vi "Teleop.vi"(10 "Match Info":T2={"Autonomous Elapsed Seconds"=0.0, "TeleOp Elapsed Seconds"=0.0, "Disabled Elapsed Seconds"=0.0, "Visited Autonomous"=FALSE, "Visited TeleOp"=FALSE, "Visited Disabled"=FALSE, "Autonomous Settings"={"Autonomous Style"=enum."Independent", "VI Refnum"=refnum}}, 11 "Call Context":T3) -> ()   [LabVIEW 2014]
doc: "This VI is called for each TeleOp packet received from the DS where the robot is not disabled. It is often used to read from the joysticks and update I/O or to update setpoints for timed control loops. It should complete and return within 20 milliseconds or it may miss DS packets."
uses:
  <vilib>/Rock Robotics/WPI/DriverStation/WPI_DriverStationDerivedRobotMode.ctl
  <vilib>/Rock Robotics/WPI/DriverStation/WPI_DriverStationMatch Info.ctl
  <vilib>/Rock Robotics/WPI/Joystick/WPI_JoystickGetSetRefNum.vi
  <vilib>/Rock Robotics/Network Tables/SD Write Boolean.vi
  <vilib>/Rock Robotics/Network Tables/SD Write Numeric Array.vi
  <vilib>/Rock Robotics/Network Tables/SD Read Boolean.vi
  <vilib>/Rock Robotics/Network Tables/SD Read Number.vi
  <vilib>/Utility/file.llb/Write To Spreadsheet File (DBL).vi
  <vilib>/Rock Robotics/WPI/RobotDrive/WPI_RobotDriveGetSetRefNum.vi
  <vilib>/Rock Robotics/WPI/RobotDrive/WPI_RobotDriveArcadeDrive_Standard(NoSaturation).vi
panel:
  in  "Claw Opened Limit":bool
  in  "Claw Closed Limit":bool
  in  "Bottom Limit":bool
  in  "Top Limit":bool
  in  "Button b":bool
  in  "Button a":bool
  in  "point reached":bool
  out "Time For Manipulator":dbl
  in  "Button y":bool
  in  "Button x":bool
  in  "Manipulator State":T1(ring)
  out "error out 2":errorcluster
  out "current (A)":dbl
  out "all currents (A)":dbl[](array[numeric])
  out "Power (W)":dbl
  out "error out 5":errorcluster
  out "error out":errorcluster
  out "Motor Values":dbl[](array[numeric])
  out "Buttons":bool[](array[boolean])
  out "Sample Slider 0":dbl(slide) scale=0.0..5.0
  out "Sample Boolean 1":bool
  out "Sample Boolean 0":bool
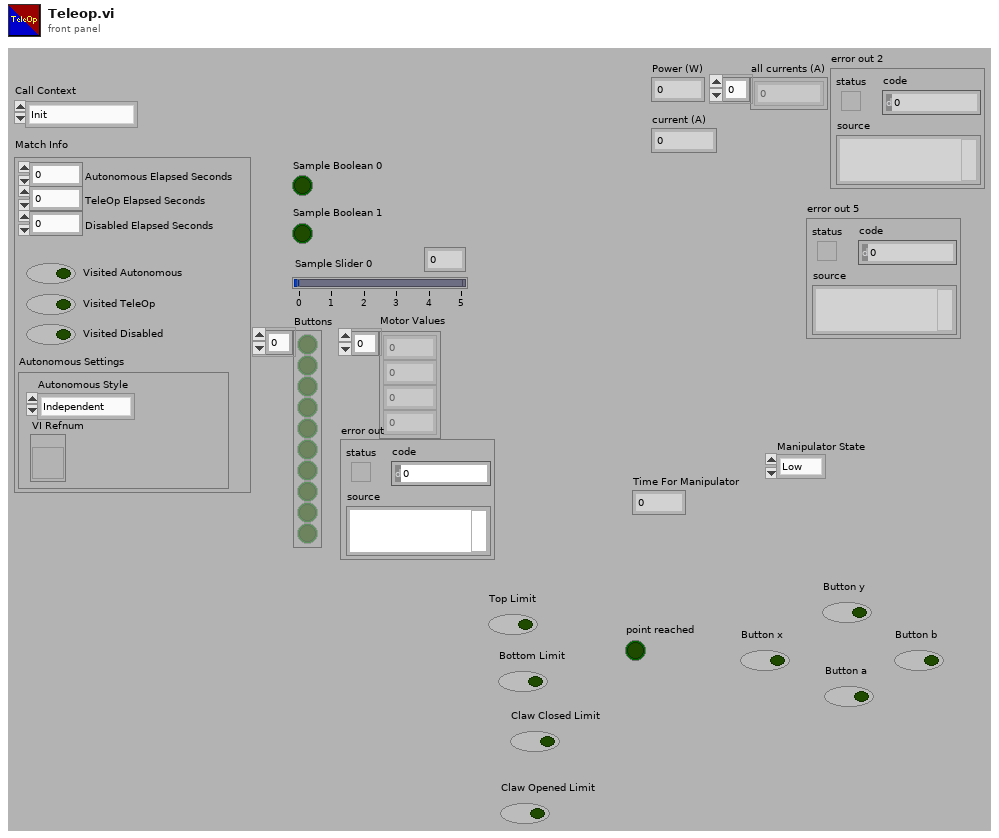
[diagram p1: front panel]
types:
  T1 = enum16{"Low", "RC Close", "Tote Close", "RC High", "Tote High", "Lowering", "Opening", "RC Top Stacker", "Bottom Stacking", "RC raising", "Tote Raising", "Limit High"}
  T2 = typedef "WPI_DriverStationMatch Info.ctl" = cluster{"Autonomous Elapsed Seconds":dbl, "TeleOp Elapsed Seconds":dbl, "Disabled Elapsed Seconds":dbl, "Visited Autonomous":bool, "Visited TeleOp":bool, "Visited Disabled":bool, "Autonomous Settings":cluster{"Autonomous Style":enum16{"Iterative", "Independent"}, "VI Refnum":refnum<vi>}}
  T3 = typedef "WPI_DriverStationDerivedRobotMode.ctl" = enum16{"Init", "Execute", "Stop"}
  T4 = typedef "WPI_RobotDriveDevRef.ctl" = cluster{"DevStatus":errorcluster, "Motors[]":T5[], "Square Inputs":bool, "Max Output":dbl}
  T5 = typedef "WPI_MotorControlDeviceRef.ctl" = cluster{"DeviceStatus":errorcluster, "Type":T6, "PWM":cluster{"Controller":T7, "PWM Channel":T8, "DeadBand":T9}, "CAN":cluster{"Device Number":u8, "Control Mode":T10, "Semaphore":T11, "Max Vout":dbl, "TalonSRX Control Mode":T12}, "Invert":bool, "TransformRef":T13, "InvTransformRef":T13}
  T6 = typedef "WPI_MotorControlType.ctl" = enum16{"PWM", "CAN", "CANTalonSRX"}
  T7 = typedef "FPGA_TypedefDigitalModule.ctl" = enum16{"Controller 1"}
  T8 = typedef "FPGA_DIOPWMChannel.ctl" = enum8{"PWM 0", "PWM 1", "PWM 2", "PWM 3", "PWM 4", "PWM 5", "PWM 6", "PWM 7", "PWM 8", "PWM 9", "PWM MXP 0", "PWM MXP 1", "PWM MXP 2", "PWM MXP 3", "PWM MXP 4", "PWM MXP 5", "PWM MXP 6", "PWM MXP 7", "PWM MXP 8", "PWM MXP 9", "Invalid"}
  T9 = typedef "WPI_PWMDeadband.ctl" = cluster{"Name":string, "maxPositivePwm":i32, "minPositivePwm":i32, "centerPwm":i32, "maxNegativePwm":i32, "minNegativePwm":i32, "angularRange":u16}
  T10 = typedef "WPI_CANJaguar_ControlMode.ctl" = enum8{"Percent VBus", "Current", "Speed", "Position", "Voltage"}
  T11 = typedef "Semaphore RefNum" = refnum<k1>
  T12 = typedef "WPI_CANTalonSRX_APIControlMode.ctl" = enum8{"Percent VBus", "Speed", "Position", "Slave", "Unchanged / Invalid"}
  T13 = typedef "WPI_PWMTransform_ConPane.ctl" = refnum<vi>
  T14 = typedef "WPI_JoystickDevRef.ctl" = cluster{"Device":T15}
  T15 = typedef "WPI_JoystickDeviceEnum.ctl" = enum16{"USB 0", "USB 1", "USB 2", "USB 3", "USB 4", "USB 5"}
  T16 = enum16{"Low", "RC Close", "Tote Close", "RC High", "Tote High", "Lowering", "Opening", "RC Top Stacker", "Bottom Stacking"}
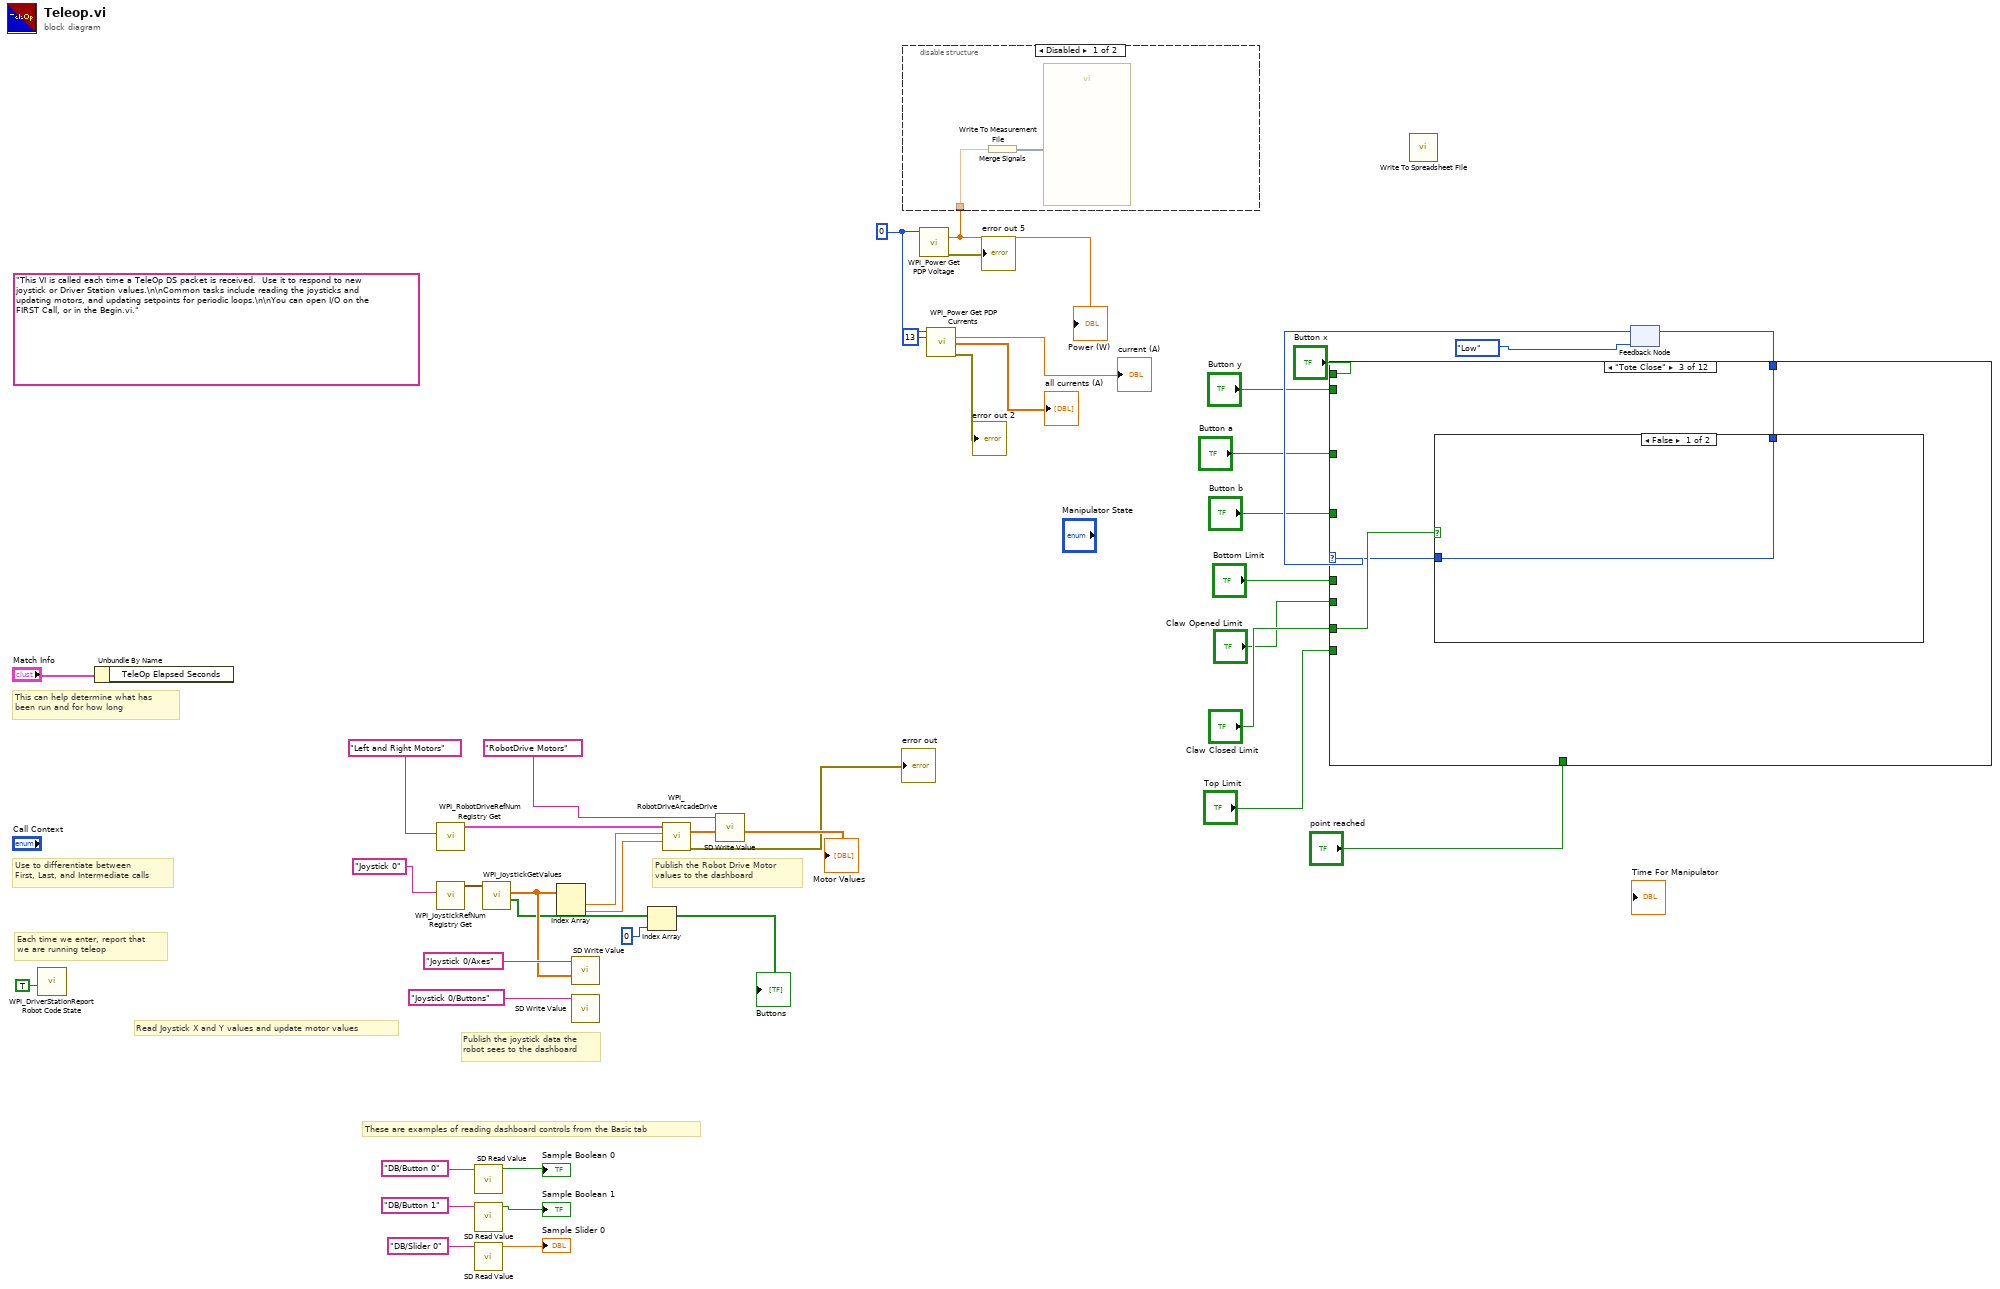
[diagram p0: block diagram]
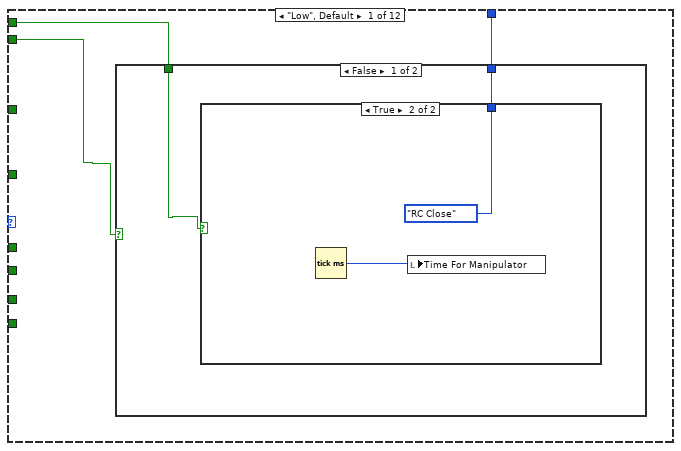
[diagram p2: hidden frame]
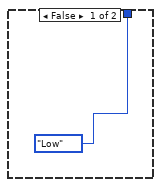
[diagram p3: hidden frame]
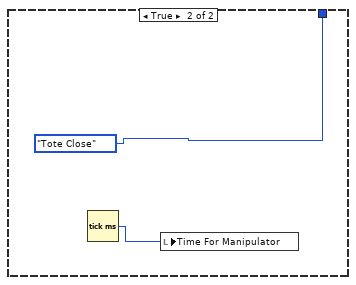
[diagram p4: hidden frame]
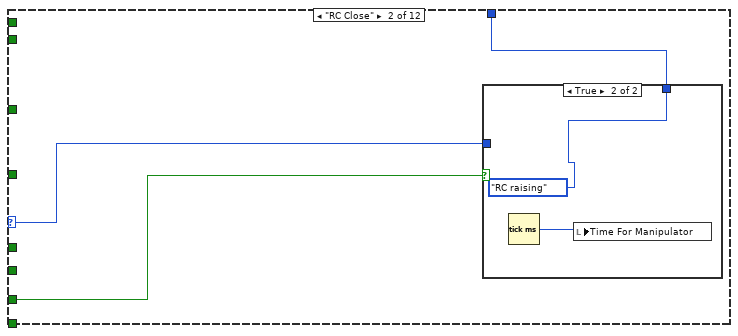
[diagram p5: hidden frame]
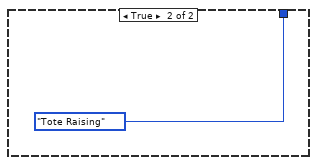
[diagram p7: hidden frame]
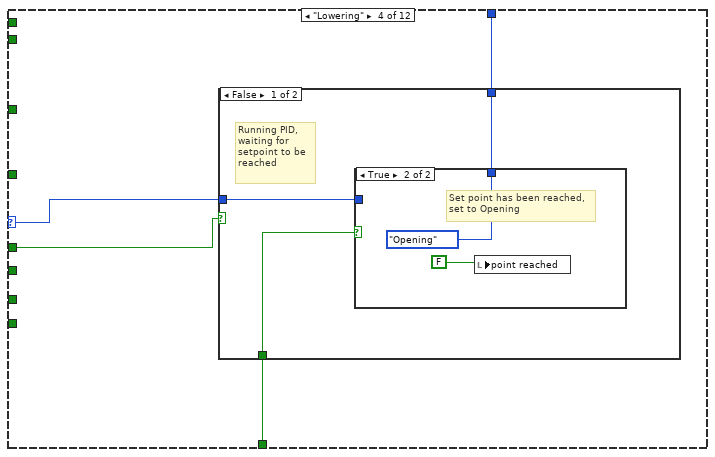
[diagram p8: hidden frame]
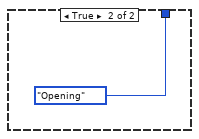
[diagram p10: hidden frame]
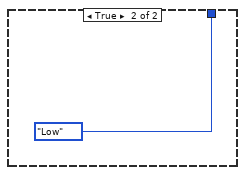
[diagram p12: hidden frame]
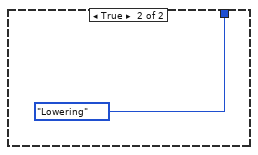
[diagram p14: hidden frame]
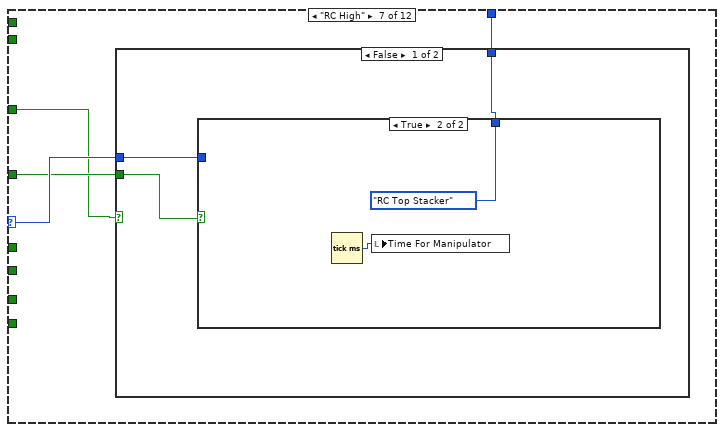
[diagram p15: hidden frame]
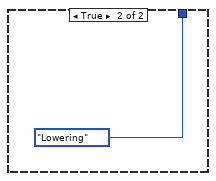
[diagram p17: hidden frame]
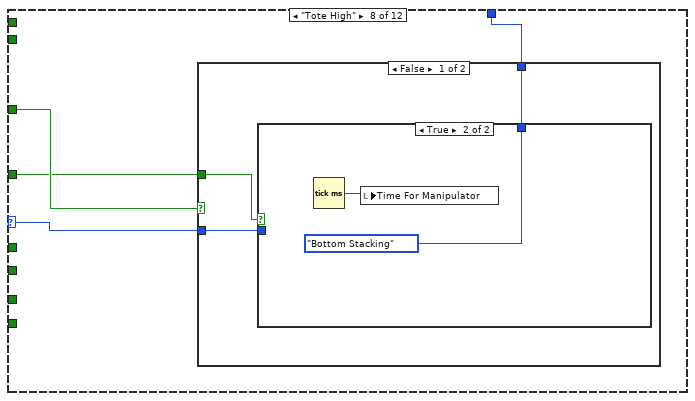
[diagram p18: hidden frame]
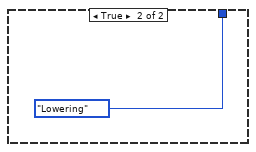
[diagram p20: hidden frame]
diagram:
  w17 = u8 0 ("Power Distribution Panel (0)")
  (unwired) "This VI is called each time a TeleOp DS packet is received.  Use it to respond to new joystick or Driver Station values.\n\nCommon tasks include reading the joysticks and updating motors, and updating setpoints for periodic loops.\n\nYou can open I/O on the FIRST Call, or in the Begin.vi."
  # "These are examples of reading dashboard controls from the Basic tab"
  # "Publish the Robot Drive Motor\nvalues to the dashboard"
  # "Publish the joystick data the\nrobot sees to the dashboard"
  # "Each time we enter, report that\nwe are running teleop"
  # "Use to differentiate between\nFirst, Last, and Intermediate calls"
  # "This can help determine what has\nbeen run and for how long"
  # "Read Joystick X and Y values and update motor values"
  n1 = call <vilib>:"WPI_DriverStationReport Robot Code State.vi"("TeleOp"=TRUE ("Autonomous")) -> ()  [unwired: 10 in, 1 out]
  n2 = Unbundle By Name("Match Info") -> ()  [unwired: 1 out]
  n3 = call <vilib>:"WPI_RobotDriveRefNum Registry Get.vi"("refnum name"="Left and Right Motors") -> ("RobotDriveDevRef"=w39:T4)  [unwired: 1 in, 9 out]
  n4 = call <vilib>:"WPI_JoystickRefNum Registry Get.vi"("refnum name"="Joystick 0") -> ("JoystickDevRef"=w36:T14)  [unwired: 1 in, 9 out]
  n5 = call-poly <vilib>:"SD Read Value.vi"("Name"="DB/Button 0" ("refnum name")) -> ("Boolean"=→"Sample Boolean 0":bool)  [unwired: 8 in, 2 out]
  n6 = call-poly <vilib>:"SD Read Value.vi"("Name"="DB/Button 1" ("refnum name")) -> ("Boolean"=→"Sample Boolean 1":bool)  [unwired: 8 in, 2 out]
  n7 = call-poly <vilib>:"SD Read Value.vi"("Name"="DB/Slider 0" ("refnum name")) -> ("Numeric"=→"Sample Slider 0":dbl)  [unwired: 8 in, 2 out]
  n8 = call <vilib>:"WPI_JoystickGetValues.vi"("JoystickDevRef"=w36) -> ("Buttons"=w23:bool[], "Axes"=w25:dbl[])  [unwired: 6 in, 3 out]
  "Buttons" <- w23
  n9 = Index Array(array=w25) -> (element #1=w38:dbl, element #2=w27:dbl)  [unwired: 2 in]
  n10 = call-poly <vilib>:"SD Write Value.vi"("Numeric Array"=w25, "Name"="Joystick 0/Axes") -> ()  [unwired: 8 in, 2 out]
  n11 = call-poly <vilib>:"SD Write Value.vi"("Name"="Joystick 0/Buttons") -> ()  [unwired: 9 in, 2 out]
  n12 = Index Array(array=w23, index=0) -> ()  [unwired: 1 out]
  n13 = call-poly <vilib>:"WPI_RobotDriveArcadeDrive.vi"("Y axis value"=w27, "X axis value"=w38, "RobotDriveDevRef"=w39) -> ("error out"=→"error out":errorcluster, "Motor Values"=w21:dbl[])  [unwired: 6 in, 1 out]
  "Motor Values" <- w21
  n14 = call-poly <vilib>:"SD Write Value.vi"("Numeric Array"=w21, "Name"="RobotDrive Motors") -> ()  [unwired: 8 in, 2 out]
  n15 = call <vilib>:"WPI_Power Get PDP Voltage.vi"("Power Distribution Panel (0)"=w17) -> ("voltage (V)"=w19:dbl, "error out"=→"error out 5":errorcluster)  [unwired: 13 in]
  "Power (W)" <- w19
  n16 = disable-structure shown="Disabled" {
    disable-tunnel: w19 -> [w43 _]
    frame Disabled {
      n17 = Merge Signals(w43) -> (w42:dynamicdata)
      n18 = call "Write To Measurement File"("Signals"=w42) -> ()  [unwired: 16 in, 3 out]
    }
    frame Enabled {
    }
  }
  n19 = call <vilib>:"WPI_Power Get PDP Currents.vi"("Power Distribution Panel (0)"=w17, "PDP Channel"=13) -> ("current (A)"=→"current (A)":dbl, "all currents (A)"=→"all currents (A)":dbl[], "error out"=→"error out 2":errorcluster)  [unwired: 11 in]
  n20 = call-poly <vilib>:"Write To Spreadsheet File.vi"() -> ()  [unwired: 8 in, 1 out]
  n21 = feedback #1(T1."Low" ("Manipulator State")) -> (w12:T1)
  n22 = case shown="\"Tote Close\"" w12 {
    selector: w12 -> [_ w55 w60 w65 w76 w81 w89 w99 w108 w117 w128 w137]
    tunnel: [w46 w56 w61 w67 w77 w82 w88 w100 w109 w119 w129 w138] -> w11
    tunnel: "Top Limit" -> [_ _ _ _ _ _ _ _ _ _ w127 w140]
    tunnel: "Bottom Limit" -> [_ _ _ w68 _ _ _ _ _ _ _ _]
    tunnel: "point reached" -> [_ _ _ w66 _ _ _ _ _ _ w126 w139]
    tunnel: "Button b" -> [_ _ _ _ _ _ w87 w97 _ _ _ _]
    tunnel: "Button a" -> [_ _ _ _ _ w83 w86 w98 _ _ _ _]
    tunnel: "Button y" -> [w45 _ _ _ _ _ _ _ _ _ _ _]
    tunnel: "Button x" -> [w44 _ _ _ _ _ _ _ _ _ _ _]
    tunnel: "Claw Closed Limit" -> [_ w54 w62 _ _ _ _ _ _ _ _ _]
    tunnel: "Claw Opened Limit" -> [_ _ _ _ w78 _ _ _ _ _ _ _]
    frame "Low", Default {
      n23 = case shown="False" w45 {
        tunnel: [w48 T1."Tote Close" ("Manipulator State")] -> w46
        tunnel: w44 -> [w47 _]
        frame False {
          n24 = case shown="True" w47 {
            tunnel: [T16."Low" ("Manipulator State") T16."RC Close" ("Manipulator State")] -> w48
            frame False {
            }
            frame True {
              n25 = Tick Count (ms)() -> (millisecond timer value=w50:u32)
              n26 = local write "Time For Manipulator"(w50) -> ()
            }
          }
        }
        frame True {
          n27 = Tick Count (ms)() -> (millisecond timer value=w53:u32)
          n28 = local write "Time For Manipulator"(w53) -> ()
        }
      }
    }
    frame "RC Close" {
      n29 = case shown="True" w54 {
        tunnel: [w57 T1."RC raising" ("Manipulator State")] -> w56
        tunnel: w55 -> [w57 _]
        frame False {
        }
        frame True {
          n30 = Tick Count (ms)() -> (millisecond timer value=w59:u32)
          n31 = local write "Time For Manipulator"(w59) -> ()
        }
      }
    }
    frame "Tote Close" {
      n32 = case shown="False" w62 {
        tunnel: [w63 T1."Tote Raising" ("Manipulator State")] -> w61
        tunnel: w60 -> [w63 _]
        frame False {
        }
        frame True {
        }
      }
    }
    frame "Lowering" {
      n33 = case shown="False" w68 {
        tunnel: [w70 T1."Opening" ("Manipulator State")] -> w67
        tunnel: w66 -> [w71 _]
        tunnel: w65 -> [w69 _]
        frame False {
          # "Running PID,\nwaiting for \nsetpoint to be \nreached"
          n34 = case shown="True" w71 {
            tunnel: [w72 T1."Opening" ("Manipulator State")] -> w70
            tunnel: w69 -> [w72 _]
            frame False {
            }
            frame True {
              # "Set point has been reached,\nset to Opening"
              n35 = local write "point reached"(FALSE) -> ()
            }
          }
        }
        frame True {
        }
      }
    }
    frame "Opening" {
      n36 = case shown="False" w78 {
        tunnel: [w79 T1."Low" ("Manipulator State")] -> w77
        tunnel: w76 -> [w79 _]
        frame False {
          # "Set Claw Motor To open at half speed"
        }
        frame True {
        }
      }
    }
    frame "Limit High" {
      n37 = case shown="False" w83 {
        tunnel: [w84 T1."Lowering" ("Manipulator State")] -> w82
        tunnel: w81 -> [w84 _]
        frame False {
        }
        frame True {
        }
      }
    }
    frame "RC High" {
      n38 = case shown="False" w86 {
        tunnel: w89 -> [w92 _]
        tunnel: [w91 T1."Lowering" ("Manipulator State")] -> w88
        tunnel: w87 -> [w90 _]
        frame False {
          n39 = case shown="True" w90 {
            tunnel: [w93 T1."RC Top Stacker" ("Manipulator State")] -> w91
            tunnel: w92 -> [w93 _]
            frame False {
            }
            frame True {
              n40 = Tick Count (ms)() -> (millisecond timer value=w94:u32)
              n41 = local write "Time For Manipulator"(w94) -> ()
            }
          }
        }
        frame True {
        }
      }
    }
    frame "Tote High" {
      n42 = case shown="False" w98 {
        tunnel: [w103 T1."Lowering" ("Manipulator State")] -> w100
        tunnel: w99 -> [w102 _]
        tunnel: w97 -> [w101 _]
        frame False {
          n43 = case shown="True" w101 {
            tunnel: [w104 T1."Bottom Stacking" ("Manipulator State")] -> w103
            tunnel: w102 -> [w104 _]
            frame False {
            }
            frame True {
              n44 = Tick Count (ms)() -> (millisecond timer value=w105:u32)
              n45 = local write "Time For Manipulator"(w105) -> ()
            }
          }
        }
        frame True {
        }
      }
    }
    frame "RC Top Stacker" {
      # "This may also include \nbacking up from the completed stack"
      # "Placing RC bin on top of stack, \n1500 ms delay symbolizes this\nfor the sake of this theoretical\nprogram"
      n46 = local read "Time For Manipulator"() -> (w113:dbl)
      n47 = Tick Count (ms)() -> (millisecond timer value=w111:u32)
      n48 = Add(x=1500.0, y=w113) -> (x+y=w112:dbl)
      n49 = Less Or Equal?(x=w112, y=w111) -> (x <= y?=w110:bool)
      n50 = case shown="True" w110 {
        tunnel: [w115 T1."Lowering" ("Manipulator State")] -> w109
        tunnel: w108 -> [w115 _]
        frame False {
        }
        frame True {
        }
      }
    }
    frame "Bottom Stacking" {
      # "This may also include \nbacking up from the completed stack"
      # "Placing RC bin on top of stack, \n1500 ms delay symbolizes this\nfor the sake of this theoretical\nprogram"
      n51 = local read "Time For Manipulator"() -> (w118:dbl)
      n52 = Tick Count (ms)() -> (millisecond timer value=w121:u32)
      n53 = Add(x=1500.0, y=w118) -> (x+y=w122:dbl)
      n54 = Less Or Equal?(x=w122, y=w121) -> (x <= y?=w120:bool)
      n55 = case shown="True" w120 {
        tunnel: [w124 T1."Lowering" ("Manipulator State")] -> w119
        tunnel: w117 -> [w124 _]
        frame False {
        }
        frame True {
        }
      }
    }
    frame "RC raising" {
      n56 = case shown="False" w127 {
        tunnel: [w132 T1."Limit High" ("Manipulator State")] -> w129
        tunnel: w128 -> [w131 _]
        tunnel: w126 -> [w130 _]
        frame False {
          # "Set Point of Manipulator PID\nto height of 'RC high', point\nreached is true when set point \nis reached."
          n57 = case shown="True" w130 {
            tunnel: [w133 T1."RC High" ("Manipulator State")] -> w132
            tunnel: w131 -> [w133 _]
            frame False {
            }
            frame True {
              n58 = local write "point reached"(FALSE) -> ()
            }
          }
        }
        frame True {
        }
      }
    }
    frame "Tote Raising" {
      n59 = case shown="False" w140 {
        tunnel: w139 -> [w143 _]
        tunnel: [w142 T1."Limit High" ("Manipulator State")] -> w138
        tunnel: w137 -> [w141 _]
        frame False {
          n60 = case shown="True" w143 {
            tunnel: [w144 T1."Tote High" ("Manipulator State")] -> w142
            tunnel: w141 -> [w144 _]
            frame False {
            }
            frame True {
            }
          }
        }
        frame True {
        }
      }
    }
  }
  n61 = feedback-in #1(w11) -> ()
